vi "test-swerve-drive-kinematics-11.vi"() -> (3 "Test Passed":bool)   [LabVIEW 2019]
uses:
  <vilib>/Rock Robotics/WPI/ThirdParty/JAS_Junk/TrajLib/Conv_Deg_Radians.vi
  <vilib>/Rock Robotics/WPI/ThirdParty/JAS_Junk/TrajLib/Rotation_CreateAngle.vi
  <vilib>/Rock Robotics/WPI/ThirdParty/JAS_Junk/TrajLib/Trajectory_Library.lvlib
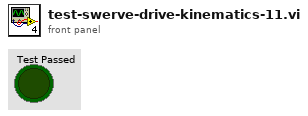
[diagram p1: front panel]
types:
  T1 = typedef "Trajectory_Library.lvlib/ROTATION2D.ctl" = cluster{"VALUE":dbl, "COS":dbl, "SIN":dbl}
  T2 = typedef "Trajectory_Library.lvlib/SWERVE_DRIVE_MODULE_STATE.ctl" = cluster{"Speed":dbl, "Angle":T1}
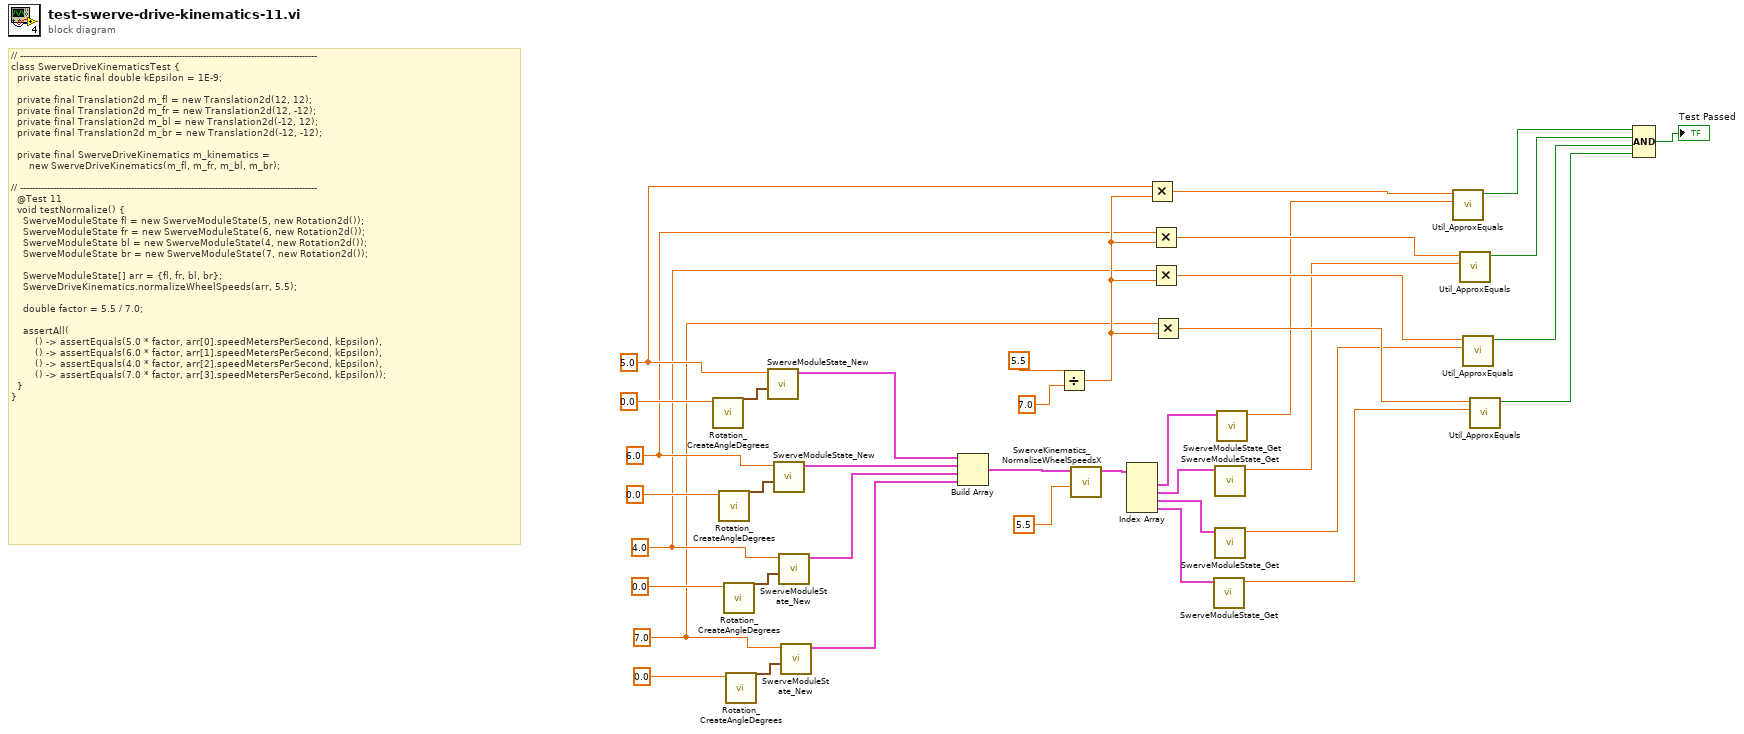
[diagram p0: block diagram]
diagram:
  w11 = 7.0 ("Speed")
  w12 = 4.0 ("Speed")
  w13 = 6.0 ("Speed")
  w14 = 5.0 ("Speed")
  # "// ---------------------------------------------------------------------------------------------------\nclass SwerveDriveKinematicsTest {\n  private static final double kEpsilon = 1E-9;\n\n  private final Translation2d m_fl = new Translation2d(12, 12);\n  private final Translation2d m_fr = new Translation2d(12, -12);\n  private final Translation2d m_bl = new Translation2d(-12, 12);\n  private final Translation2d m_br = new Translation2d(-12, -12);\n\n  private final SwerveDriveKinematics m_kinematics =\n      new SwerveDriveKinematics(m_fl, m_fr, m_bl, m_br);\n\n// ---------------------------------------------------------------------------------------------------\n  @Test 11\n  void testNormalize() {\n    SwerveModuleState fl = new SwerveModuleState(5, new Rotation2d());\n    SwerveModuleState fr = new SwerveModuleState(6, new Rotation2d());\n    SwerveModuleState bl = new SwerveModuleState(4, new Rotation2d());\n    SwerveModuleState br = new SwerveModuleState(7, new Rotation2d());\n\n    SwerveModuleState[] arr = {fl, fr, bl, br};\n    SwerveDriveKinematics.normalizeWheelSpeeds(arr, 5.5);\n\n    double factor = 5.5 / 7.0;\n\n    assertAll(\n        () -> assertEquals(5.0 * factor, arr[0].speedMetersPerSecond, kEpsilon),\n        () -> assertEquals(6.0 * factor, arr[1].speedMetersPerSecond, kEpsilon),\n        () -> assertEquals(4.0 * factor, arr[2].speedMetersPerSecond, kEpsilon),\n        () -> assertEquals(7.0 * factor, arr[3].speedMetersPerSecond, kEpsilon));\n  }\n}"
  n1 = call <vilib>:"Rotation_CreateAngleDegrees.vi"("Angle_Degrees"=0.0) -> ("ROTATION"=w36:T1)  [unwired: 10 in]
  n2 = call <vilib>:"Rotation_CreateAngleDegrees.vi"("Angle_Degrees"=0.0) -> ("ROTATION"=w34:T1)  [unwired: 10 in]
  n3 = call <vilib>:"Rotation_CreateAngleDegrees.vi"("Angle_Degrees"=0.0) -> ("ROTATION"=w32:T1)  [unwired: 10 in]
  n4 = call <vilib>:"Rotation_CreateAngleDegrees.vi"("Angle_Degrees"=0.0) -> ("ROTATION"=w30:T1)  [unwired: 10 in]
  n5 = call <vilib>:"SwerveModuleState_New.vi"("ROTATION"=w36, "Speed"=w14) -> ("SWERVE_DRIVE_MODULE_STATE"=w26:T2)  [unwired: 9 in]
  n6 = call <vilib>:"SwerveModuleState_New.vi"("ROTATION"=w34, "Speed"=w13) -> ("SWERVE_DRIVE_MODULE_STATE"=w25:T2)  [unwired: 9 in]
  n7 = call <vilib>:"SwerveModuleState_New.vi"("ROTATION"=w32, "Speed"=w12) -> ("SWERVE_DRIVE_MODULE_STATE"=w24:T2)  [unwired: 9 in]
  n8 = call <vilib>:"SwerveModuleState_New.vi"("ROTATION"=w30, "Speed"=w11) -> ("SWERVE_DRIVE_MODULE_STATE"=w23:T2)  [unwired: 9 in]
  n9 = Build Array(w26, w25, w24, w23) -> (w27:T2[])
  n10 = Divide(x=5.5, y=7.0) -> (x/y=w15:dbl)
  n11 = call <vilib>:"SwerveKinematics_NormalizeWheelSpeedsX.vi"("AttainableMaxSpeed"=5.5, "in WheelStates"=w27) -> ("out WheelStates"=w20:T2[])  [unwired: 9 in]
  n12 = Index Array(array=w20) -> (element #1=w19:T2, element #2=w18:T2, element #3=w17:T2, element #4=w16:T2)  [unwired: 4 in]
  n13 = Multiply(x=w14, y=w15) -> (x*y=w8:dbl)
  n14 = Multiply(x=w13, y=w15) -> (x*y=w7:dbl)
  n15 = Multiply(x=w12, y=w15) -> (x*y=w6:dbl)
  n16 = Multiply(x=w11, y=w15) -> (x*y=w5:dbl)
  n17 = call <vilib>:"SwerveModuleState_Get.vi"("Desired State"=w16) -> ("Speed M/S"=w1:dbl)  [unwired: 9 in, 1 out]
  n18 = call <vilib>:"SwerveModuleState_Get.vi"("Desired State"=w18) -> ("Speed M/S"=w3:dbl)  [unwired: 9 in, 1 out]
  n19 = call <vilib>:"SwerveModuleState_Get.vi"("Desired State"=w17) -> ("Speed M/S"=w2:dbl)  [unwired: 9 in, 1 out]
  n20 = call <vilib>:"SwerveModuleState_Get.vi"("Desired State"=w19) -> ("Speed M/S"=w4:dbl)  [unwired: 9 in, 1 out]
  n21 = call <vilib>:"Util_ApproxEquals.vi"("Value 2"=w4, "Value 1"=w8) -> ("ApproxEquals"=w39:bool)  [unwired: 9 in]
  n22 = call <vilib>:"Util_ApproxEquals.vi"("Value 2"=w3, "Value 1"=w7) -> ("ApproxEquals"=w38:bool)  [unwired: 9 in]
  n23 = call <vilib>:"Util_ApproxEquals.vi"("Value 2"=w2, "Value 1"=w6) -> ("ApproxEquals"=w10:bool)  [unwired: 9 in]
  n24 = call <vilib>:"Util_ApproxEquals.vi"("Value 2"=w1, "Value 1"=w5) -> ("ApproxEquals"=w9:bool)  [unwired: 9 in]
  n25 = Compound Arithmetic op=AND(w39, w38, w10, w9) -> (→"Test Passed":bool)
